vi "final(1).vi"() -> ()   [LabVIEW 2009]
uses:
  <vilib>/Utility/file.llb/Write To Spreadsheet File (string).vi
panel:
  out "Time has Elapsed":bool
  out "Current Temp":dbl(slide) scale=0.0..100.0
  in  "stop":bool
  out "Lid (on indicates open)":bool[](array[boolean])
  out "Heating":bool[](array[boolean])
  out "Cooling":bool[](array[boolean])
  in  "Power":bool
  out "Temperature":dbl(graph)
  out "Notifications":string
  in  "Time (min)":dbl
  in  "Start":bool
  in  "High Temp":dbl
  in  "Low Temp":dbl
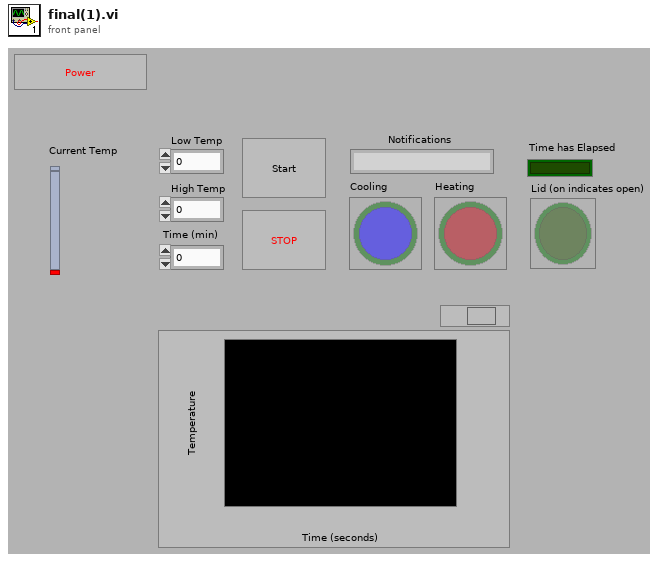
[diagram p1: front panel]
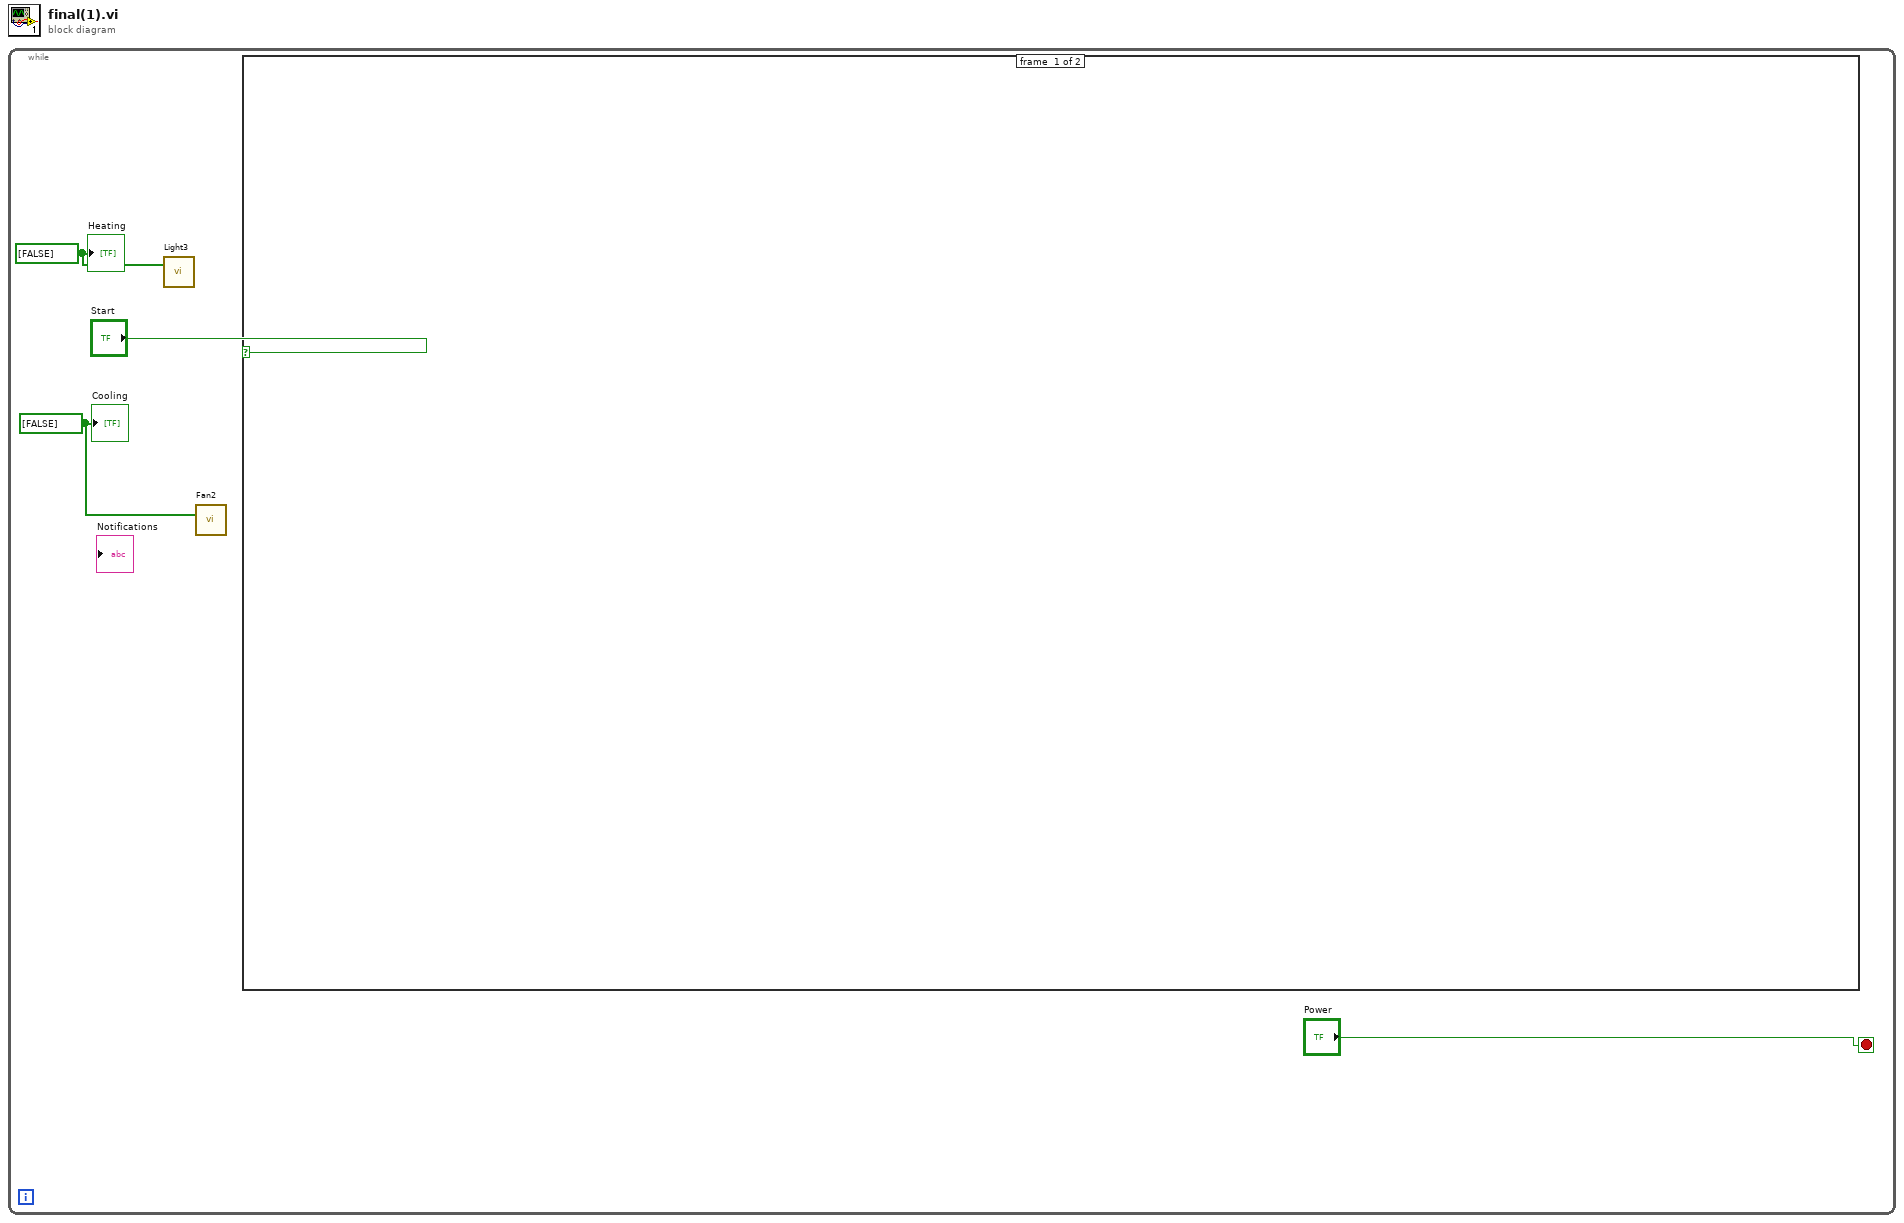
[diagram p0: block diagram]
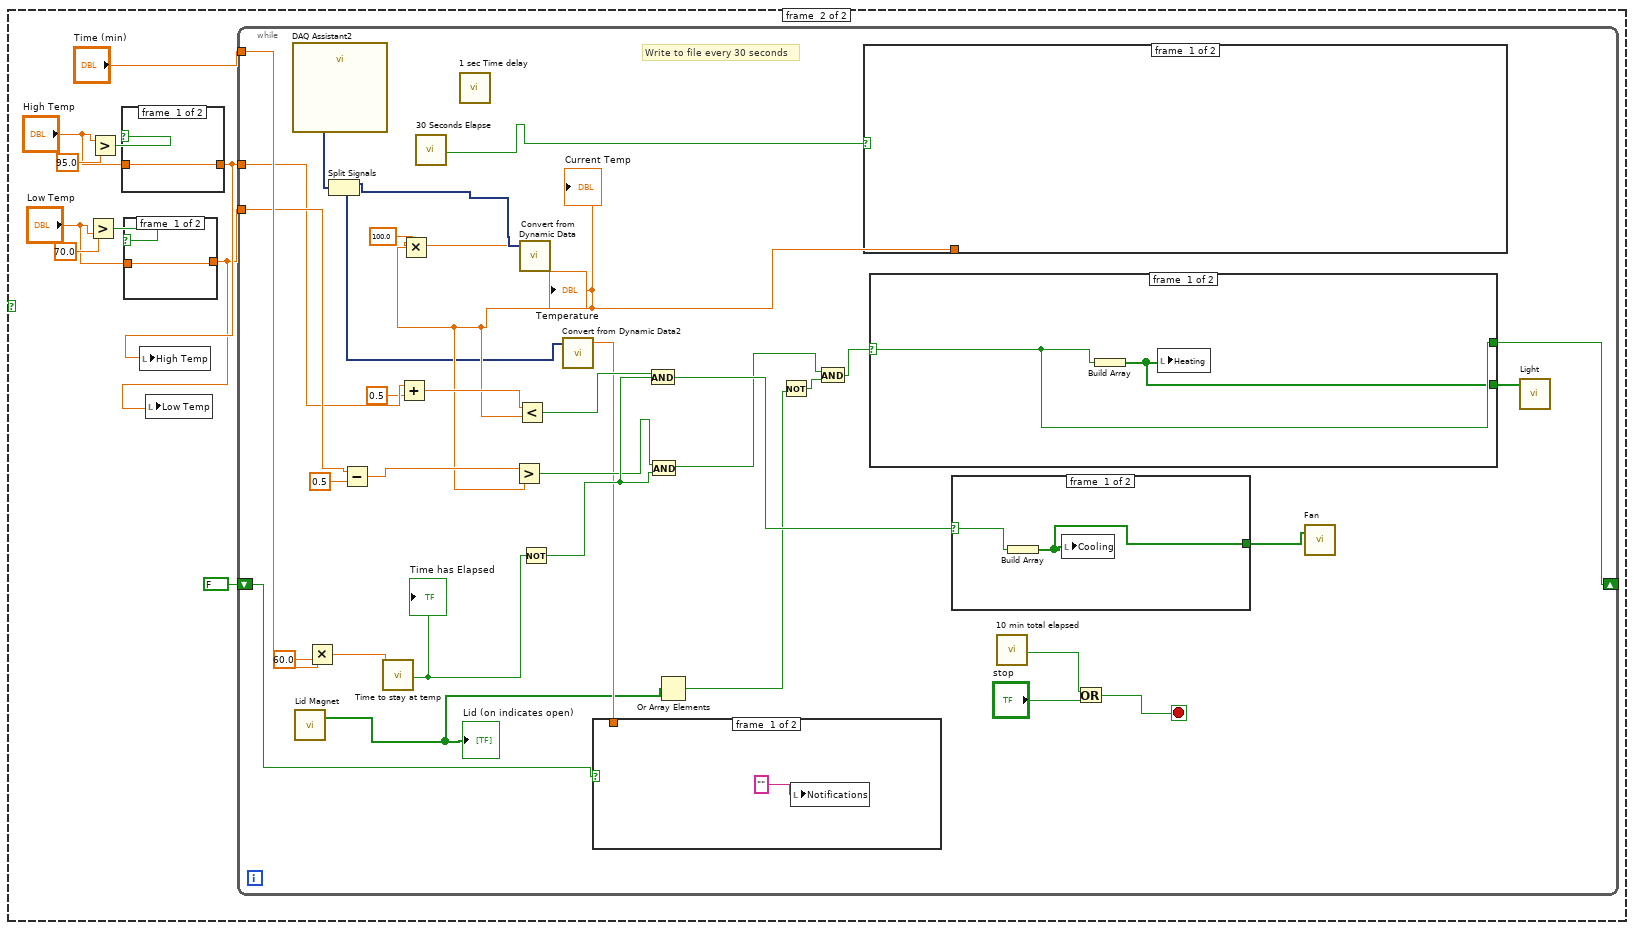
[diagram p2: hidden frame]
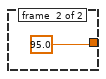
[diagram p3: hidden frame]
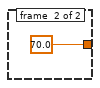
[diagram p4: hidden frame]
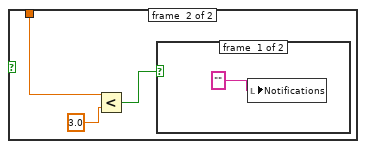
[diagram p5: hidden frame]
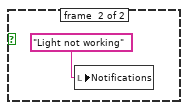
[diagram p6: hidden frame]
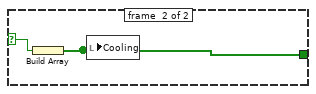
[diagram p7: hidden frame]
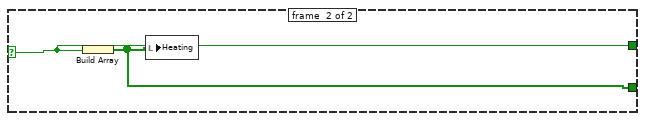
[diagram p8: hidden frame]
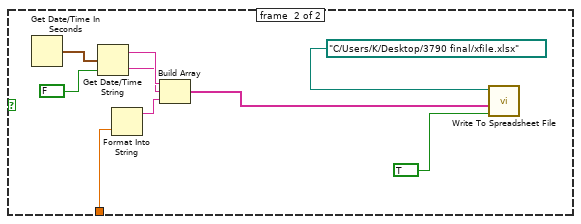
[diagram p9: hidden frame]
diagram:
  n1 = while {
    stop <- "Power" stop-if-true
    w1 = bool[] [FALSE] ("Heating")
    w2 = bool[] [FALSE] ("Cooling")
    n2 = call "Light3"("data"=w1) -> ()  [unwired: 17 in, 2 out]
    n3 = call "Fan2"("data"=w2) -> ()  [unwired: 17 in, 2 out]
    n4 = case shown="True" "Start" {
      frame #0 {
      }
      frame #1 {
        n5 = Greater?(x=70.0, y="Low Temp") -> (0:w11:bool)
        n6 = Greater?(x="High Temp", y=95.0) -> (0:w9:bool)
        n7 = case shown="False" w9 {
          tunnel: [w15 95.0 ("y")] -> w6
          tunnel: "High Temp" -> [w15 _]
          frame #0 {
          }
          frame #1 {
          }
        }
        n8 = case shown="False" w11 {
          tunnel: [w17 70.0 ("x")] -> w5
          tunnel: "Low Temp" -> [w17 _]
          frame #0 {
          }
          frame #1 {
          }
        }
        n9 = local write "High Temp"(w6) -> ()
        n10 = local write "Low Temp"(w5) -> ()
        n11 = while {
          tunnel: w6 -> [w32]
          tunnel: w5 -> [w35]
          tunnel: "Time (min)" -> [w51]
          shift-right: [w27] -> _
          shift-left: FALSE -> [w25]
          stop <- w46 stop-if-true
          # "Write to file every 30 seconds"
          n12 = call "DAQ Assistant2"() -> ("data"=w39:dynamicdata)  [unwired: 16 in, 3 out]
          n13 = call "Lid Magnet"() -> ("data"=w20:bool[])  [unwired: 17 in, 2 out]
          "Lid (on indicates open)" <- w20
          n14 = Multiply(x=w51, y=60.0) -> (x*y=w50:dbl)
          n15 = Split Signals(w39) -> (w38:dynamicdata, w28:dynamicdata)  [unwired: 2 in]
          n16 = Subtract(x=w35, y=0.5) -> (x-y=w34:dbl)
          n17 = call "Time to stay at temp"("Time Target (s)"=w50) -> ("Time has Elapsed"=w45:bool)  [unwired: 11 in, 7 out]
          "Time has Elapsed" <- w45
          n18 = Add(x=w32, y=0.5) -> (x+y=w30:dbl)
          n19 = call "30 Seconds Elapse"() -> ("Time has Elapsed"=w49:bool)  [unwired: 12 in, 7 out]
          n20 = call "1 sec Time delay"() -> ()  [unwired: 11 in, 1 out]
          n21 = call "Convert from Dynamic Data"("Dynamic Data Type"=w38) -> ("Scalar"=w37:dbl)  [unwired: 3 in]
          n22 = Multiply(x=w37, y=100.0) -> (x*y=w29:dbl)
          "Temperature" <- w29
          "Current Temp" <- w29
          n23 = Greater?(x=w34, y=w29) -> (0:w43:bool)
          n24 = Less?(x=w30, y=w29) -> (x < y?=w42:bool)
          n25 = Not(x=w45) -> (.not. x?=w44:bool)
          n26 = call "Convert from Dynamic Data2"("Dynamic Data Type"=w28) -> ("Scalar"=w26:dbl)  [unwired: 3 in]
          n27 = case shown="True" w25 {
            tunnel: w26 -> [_ w54]
            frame #0 {
              n28 = local write "Notifications"("" ("Notifications")) -> ()
            }
            frame #1 {
              n29 = Less?(x=w54, y=3.0 ("x")) -> (x < y?=w55:bool)
              n30 = case shown="True" w55 {
                frame #0 {
                  n31 = local write "Notifications"("" ("Notifications")) -> ()
                }
                frame #1 {
                  n32 = local write "Notifications"("Light not working" ("Notifications")) -> ()
                }
              }
            }
          }
          n33 = And(x=w42, y=w44) -> (x .and. y?=w36:bool)
          n34 = And(x=w43, y=w44) -> (x .and. y?=w22:bool)
          n35 = Or Array Elements(Boolean array=w20) -> (logical OR=w19:bool)
          n36 = Not(x=w19) -> (.not. x?=w23:bool)
          n37 = And(x=w22, y=w23) -> (x .and. y?=w21:bool)
          n38 = case shown="True" w49 {
            tunnel: w29 -> [_ w69]
            frame #0 {
            }
            frame #1 {
              n39 = Get Date/Time In Seconds() -> (seconds since 1Jan1904=w72:timestamp)
              n40 = Get Date/Time String(seconds (now)=w72, want seconds? (F)=FALSE) -> (date string=w68:string, time string=w67:string)  [unwired: 1 in]
              n41 = Format Into String(w69) -> (resulting string=w70:string)  [unwired: 3 in, 1 out]
              n42 = Build Array(w68, w67, w70) -> (w73:string[])
              n43 = call-poly <vilib>:"Write To Spreadsheet File.vi"("append to file? (new file:F)"=TRUE, "1D data"=w73, "file path (dialog if empty)"=path "C:/Users/K/Desktop/3790 final/xfile.xlsx") -> ()  [unwired: 5 in, 1 out]
            }
          }
          n44 = case shown="True" w21 {
            selector: w21 -> [w64 w66]
            tunnel: [w64 w66] -> w27
            tunnel: [w63 w65] -> w24
            frame #0 {
              n45 = Build Array(w64) -> (w63:bool[])
              n46 = local write "Heating"(w63) -> ()
            }
            frame #1 {
              n47 = Build Array(w66) -> (w65:bool[])
              n48 = local write "Heating"(w65) -> ()
            }
          }
          n49 = case shown="False" w36 {
            selector: w36 -> [w60 w62]
            tunnel: [w59 w61] -> w41
            frame #0 {
              n50 = Build Array(w60) -> (w59:bool[])
              n51 = local write "Cooling"(w59) -> ()
            }
            frame #1 {
              n52 = Build Array(w62) -> (w61:bool[])
              n53 = local write "Cooling"(w61) -> ()
            }
          }
          n54 = call "10 min total elapsed"() -> ("Time has Elapsed"=w47:bool)  [unwired: 12 in, 7 out]
          n55 = Or(x=w47, y="stop") -> (x .or. y?=w46:bool)
          n56 = call "Fan"("data"=w41) -> ()  [unwired: 17 in, 2 out]
          n57 = call "Light"("data"=w24) -> ()  [unwired: 17 in, 2 out]
        }
      }
    }
    "Heating" <- w1
    "Cooling" <- w2
  }
